vi "FTW-Test-SQLite-FloatingPoint.vi"() -> (0 "Test Result":errorcluster)   [LabVIEW 2015]
uses:
  src/database/core/FTW-SQLite-Core-PrepareStatement.vi
  src/database/core/FTW-SQLite-Core-LibraryReturnValue.vi
  src/error/FTW-ERR-Assert-DeveloperError.vi
  src/error/FTW-ERR-StatusOK.vi
  src/database/core/FTW-SQLite-Core-QueryDebug.vi
  codegen/xnode/FTW-SQLite-Insert.xnode
  src/core/type/FTW-Type-SQLite.ctl
  codegen/xnode/FTW-SQLite-Fetch.xnode
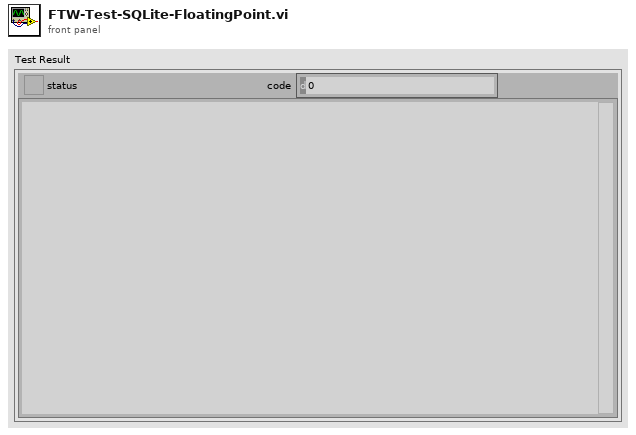
[diagram p1: front panel]
types:
  T1 = typedef "FTW-Type-SQLite.ctl" = refnum<data-value>
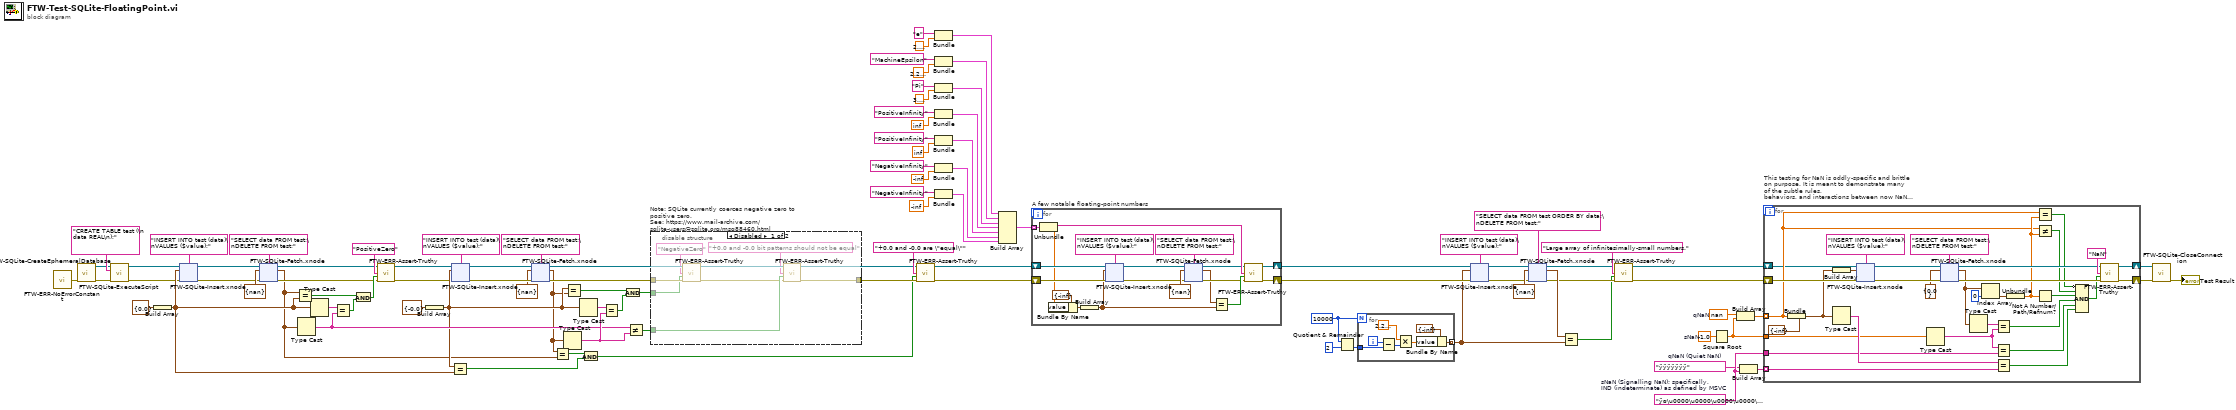
[diagram p0: block diagram]
diagram:
  w3 = 10000
  w25 = "ÿÿÿÿÿÿÿ"  # qNaN (Quiet NaN)
  w26 = "ÿø\u0000\u0000\u0000\u0000\u0000\u0000"  # sNaN (Signalling NaN); specifically, IND (indeterminate) as defined by MSVC
  w29 = -1.0  # sNaN
  w28 = nan  # qNaN
  n1 = call "FTW-ERR-NoErrorConstant.vi"() -> ("no error"=w93:errorcluster)
  n2 = call "FTW-SQLite-CreateEphemeralDatabase.vi"("error in"=w93) -> ("SQLite Connection"=w77:T1, "error out"=w76:errorcluster)  [unwired: 13 in]
  n3 = call "FTW-SQLite-ExecuteScript.vi"("SQLite Connection"=w77, "SQL Script"="CREATE TABLE test (\n    data REAL\n);", "error in"=w76) -> ("SQLite Connection out"=w39:T1, "error out"=w38:errorcluster)  [unwired: 10 in, 1 out]
  n4 = Build Array(cluster{"value":dbl} {"value"=0.0}) -> (w53:cluster{"value":dbl}[])
  n5 = xnode "FTW-SQLite-Insert.xnode"("SQLite Connection"=w39, "SQL Script"="INSERT INTO test (data)\nVALUES ($value);", "Data to Insert"=w53, "error in"=w38) -> ("SQLite Connection out"=w66:T1, "error out"=w65:errorcluster)  [unwired: 1 in, 1 out]
  n6 = xnode "FTW-SQLite-Fetch.xnode"("SQLite Connection"=w66, "SQL Script"="SELECT data FROM test;\nDELETE FROM test;", "Row Datatype"=cluster{"value":dbl} {"value"=nan}, "error in"=w65) -> ("SQLite Connection out"=w37:T1, "Result Set"=w21:cluster{"value":dbl}[], "error out"=w36:errorcluster)  [unwired: 1 out]
  n7 = Equal?(x=w21, y=w53) -> (x = y?=w56:bool)
  n8 = Type Cast(x=w21) -> (*(type *) &x=w54:string)  [unwired: 1 in]
  n9 = Type Cast(x=w53) -> (*(type *) &x=w58:string)  [unwired: 1 in]
  n10 = Equal?(x=w58, y=w54) -> (x = y?=w57:bool)
  n11 = And(x=w56, y=w57) -> (x .and. y?=w55:bool)
  n12 = call "FTW-ERR-Assert-Truthy.vi"("Assertion"="PositiveZero" ("Key"), "Assertion holds true?"=w55, "error in"=w36) -> ("error out"=w35:errorcluster)  [unwired: 12 in]
  n13 = Build Array(cluster{"value":dbl} {"value"=-0.0}) -> (w52:cluster{"value":dbl}[])
  n14 = Equal?(x=w52, y=w53) -> (x = y?=w19:bool)
  n15 = xnode "FTW-SQLite-Insert.xnode"("SQLite Connection"=w37, "SQL Script"="INSERT INTO test (data)\nVALUES ($value);", "Data to Insert"=w52, "error in"=w35) -> ("SQLite Connection out"=w73:T1, "error out"=w74:errorcluster)  [unwired: 1 in, 1 out]
  n16 = xnode "FTW-SQLite-Fetch.xnode"("SQLite Connection"=w73, "SQL Script"="SELECT data FROM test;\nDELETE FROM test;", "Row Datatype"=cluster{"value":dbl} {"value"=nan}, "error in"=w74) -> ("SQLite Connection out"=w32:T1, "Result Set"=w22:cluster{"value":dbl}[], "error out"=w34:errorcluster)  [unwired: 1 out]
  n17 = Equal?(x=w22, y=w21) -> (x = y?=w20:bool)
  n18 = Type Cast(x=w22) -> (*(type *) &x=w61:string)  [unwired: 1 in]
  n19 = Equal?(x=w52, y=w22) -> (x = y?=w59:bool)
  n20 = Type Cast(x=w52) -> (*(type *) &x=w62:string)  [unwired: 1 in]
  n21 = And(x=w20, y=w19) -> (x .and. y?=w18:bool)
  n22 = Equal?(x=w62, y=w61) -> (x = y?=w60:bool)
  n23 = And(x=w59, y=w60) -> (x .and. y?=w33:bool)
  n24 = Not Equal?(x=w54, y=w61) -> (x != y?=w89:bool)
  n25 = disable-structure "Note: SQLite currently coerces negative zero to positive zero.\nSee: https://www.mail-archive.com/sqlite-users@sqlite.org/msg88460.html" shown="Disabled" {
    disable-tunnel: [w99 w101] -> w90
    disable-tunnel: w89 -> [w98 _]
    disable-tunnel: w34 -> [w96 w101]
    disable-tunnel: w33 -> [w95 _]
    frame Disabled {
      n26 = call "FTW-ERR-Assert-Truthy.vi"("Assertion"="NegativeZero" ("Key"), "Assertion holds true?"=w95, "error in"=w96) -> ("error out"=w94:errorcluster)  [unwired: 12 in]
      n27 = call "FTW-ERR-Assert-Truthy.vi"("Assertion"="+0.0 and -0.0 bit patterns should not be equal", "Assertion holds true?"=w98, "error in"=w94) -> ("error out"=w99:errorcluster)  [unwired: 12 in]
    }
    frame Enabled {
    }
  }
  n28 = call "FTW-ERR-Assert-Truthy.vi"("Assertion"="+0.0 and -0.0 are \"equal\"", "Assertion holds true?"=w18) -> ()  [unwired: 13 in, 1 out]
  n29 = Bundle("Key"="e", 2.718281828459045) -> (w86:cluster{"Key":string, dbl})  [unwired: 1 in]
  n30 = Bundle("Key"="MachineEpsilon", 2.220446049250313e-16) -> (w82:cluster{"Key":string, dbl})  [unwired: 1 in]
  n31 = Bundle("Key"="Pi", 3.141592653589793) -> (w79:cluster{"Key":string, dbl})  [unwired: 1 in]
  n32 = Bundle("Key"="PositiveInfinity", inf) -> (w47:cluster{"Key":string, dbl})  [unwired: 1 in]
  n33 = Bundle("Key"="PositiveInfinity", "value"=inf) -> (w46:cluster{"Key":string, "value":dbl})  [unwired: 1 in]
  n34 = Bundle("Key"="NegativeInfinity", -inf) -> (w41:cluster{"Key":string, dbl})  [unwired: 1 in]
  n35 = Bundle("Key"="NegativeInfinity", "value"=-inf) -> (w40:cluster{"Key":string, "value":dbl})  [unwired: 1 in]
  n36 = Build Array(w86, w82, w79, w47, w46, w41, w40) -> (w85:cluster{"Key":string, "value":dbl}[])
  n37 = for "A few notable floating-point numbers" {
    shift-right: [w103] -> w16
    shift-left: w32 -> [w110]
    shift-right: [w102] -> w15
    shift-left: w90 -> [w111]
    tunnel: w85 -> [w119] mode=indexing
    n38 = Unbundle(w119) -> ("Key"=w109:string, "value"=w106:dbl)
    n39 = Bundle By Name(cluster=cluster{"value":dbl} {"value"=-inf}, "value"=w106) -> (w107:cluster{"value":dbl})
    n40 = Build Array(w107) -> (w105:cluster{"value":dbl}[])
    n41 = xnode "FTW-SQLite-Insert.xnode"("SQLite Connection"=w110, "SQL Script"="INSERT INTO test (data)\nVALUES ($value);", "Data to Insert"=w105, "error in"=w111) -> ("SQLite Connection out"=w114:T1, "error out"=w113:errorcluster)  [unwired: 1 in, 1 out]
    n42 = xnode "FTW-SQLite-Fetch.xnode"("SQLite Connection"=w114, "SQL Script"="SELECT data FROM test;\nDELETE FROM test;", "Row Datatype"=cluster{"value":dbl} {"value"=nan}, "error in"=w113) -> ("SQLite Connection out"=w103:T1, "Result Set"=w104:cluster{"value":dbl}[], "error out"=w117:errorcluster)  [unwired: 1 out]
    n43 = Equal?(x=w104, y=w105) -> (x = y?=w118:bool)
    n44 = call "FTW-ERR-Assert-Truthy.vi"("Assertion"=w109, "Assertion holds true?"=w118, "error in"=w117) -> ("error out"=w102:errorcluster)  [unwired: 12 in]
  }
  n45 = Quotient & Remainder(x=w3, y=2) -> (floor(x/y)=w1:i32)  [unwired: 1 out]
  n46 = for {
    N: w3 -> [_]
    tunnel: [w330] -> w5 mode=indexing
    tunnel: w1 -> [w327]
    i -> [w329]
    n47 = Subtract(x=w329, y=w327) -> (x-y=w328:i32)
    n48 = Multiply(x=2.220446049250313e-16, y=w328) -> (x*y=w331:dbl)
    n49 = Bundle By Name(cluster=cluster{"value":dbl} {"value"=-inf}, "value"=w331) -> (w330:cluster{"value":dbl})
  }
  n50 = xnode "FTW-SQLite-Insert.xnode"("SQLite Connection"=w16, "SQL Script"="INSERT INTO test (data)\nVALUES ($value);", "Data to Insert"=w5, "error in"=w15) -> ("SQLite Connection out"=w11:T1, "error out"=w12:errorcluster)  [unwired: 1 in, 1 out]
  n51 = xnode "FTW-SQLite-Fetch.xnode"("SQLite Connection"=w11, "SQL Script"="SELECT data FROM test ORDER BY data;\nDELETE FROM test;", "Row Datatype"=cluster{"value":dbl} {"value"=nan}, "error in"=w12) -> ("SQLite Connection out"=w4:T1, "Result Set"=w10:cluster{"value":dbl}[], "error out"=w9:errorcluster)  [unwired: 1 out]
  n52 = Equal?(x=w10, y=w5) -> (x = y?=w6:bool)
  n53 = call "FTW-ERR-Assert-Truthy.vi"("Assertion"="Large array of infinitesimally-small numbers.", "Assertion holds true?"=w6, "error in"=w9) -> ("error out"=w8:errorcluster)  [unwired: 12 in]
  n54 = Square Root(x=w29) -> (sqrt(x)=w23:dbl)
  n55 = Build Array(w28, w23) -> (w27:dbl[])
  n56 = Build Array(w25, w26) -> (w24:string[])
  n57 = for "This testing for NaN is oddly-specific and brittle on purpose. It is meant to demonstrate many of the subtle rules,\nbehaviors, and interactions between now NaN is defined by IEEE 754, not defined by ANSI C, yet implemented by\nLabVIEW, C and SQLite. Initially tested on WIN32, failures on additional platforms might indicate the need for\nconditional disable structures to expand these assertions based on platform." {
    shift-right: [w349] -> w30
    shift-left: w8 -> [w357]
    shift-right: [w350] -> w31
    shift-left: w4 -> [w336]
    tunnel: w27 -> [w340] mode=indexing
    tunnel: w26 -> [w343]
    tunnel: w24 -> [w342] mode=indexing
    tunnel: w23 -> [w337]
    n58 = Bundle(cluster=cluster{"value":dbl} {"value"=-inf}, "value"=w340) -> (w344:cluster{"value":dbl})
    n59 = Build Array(w344) -> (w356:cluster{"value":dbl}[])
    n60 = Type Cast(x=w344) -> (*(type *) &x=w347:string)  [unwired: 1 in]
    n61 = xnode "FTW-SQLite-Insert.xnode"("SQLite Connection"=w336, "SQL Script"="INSERT INTO test (data)\nVALUES ($value);", "Data to Insert"=w356, "error in"=w357) -> ("SQLite Connection out"=w363:T1, "error out"=w364:errorcluster)  [unwired: 1 in, 1 out]
    n62 = Type Cast(x=w337) -> (*(type *) &x=w348:string)  [unwired: 1 in]
    n63 = xnode "FTW-SQLite-Fetch.xnode"("SQLite Connection"=w363, "SQL Script"="SELECT data FROM test;\nDELETE FROM test;", "Row Datatype"=cluster{"value":dbl} {"value"=0.0}, "error in"=w364) -> ("SQLite Connection out"=w350:T1, "Result Set"=w334:cluster{"value":dbl}[], "error out"=w360:errorcluster)  [unwired: 1 out]
    n64 = Type Cast(x=w334) -> (*(type *) &x=w355:string)  [unwired: 1 in]
    n65 = Index Array(array=w334, index=0) -> (element=w354:cluster{"value":dbl})
    n66 = Equal?(x=w355, y=w348) -> (x = y?=w353:bool)
    n67 = Equal?(x=w348, y=w343) -> (x = y?=w346:bool)
    n68 = Equal?(x=w347, y=w342) -> (x = y?=w345:bool)
    n69 = Unbundle(w354) -> ("value"=w341:dbl)
    n70 = Equal?(x=w340, y=w341) -> (x = y?=w338:bool)
    n71 = Not Equal?(x=w340, y=w341) -> (x != y?=w339:bool)
    n72 = Not A Number/Path/Refnum?(number/path/refnum=w341) -> (NaN/Path/Refnum?=w352:bool)
    n73 = Compound Arithmetic op=AND(invert w338, w339, w352, w353, w346, w345) -> (w351:bool)
    n74 = call "FTW-ERR-Assert-Truthy.vi"("Assertion"="NaN" ("Key"), "Assertion holds true?"=w351, "error in"=w360) -> ("error out"=w349:errorcluster)  [unwired: 12 in]
  }
  n75 = call "FTW-SQLite-CloseConnection.vi"("SQLite Connection"=w31, "error in"=w30) -> ("error out"=→"Test Result":errorcluster)  [unwired: 13 in]
